vi "Main - Menu Button Ref FGV.vi"(7 "Action":T1=enum."Write", 8 "error In":errorcluster, 11 "Menu Button Ref In":refnum<vi>[](array[refnum])) -> (0 "error out":errorcluster, 3 "Menu Button Ref Out":refnum<vi>[](array[refnum]))   [LabVIEW 2019]
uses:
  Controls/FGV States.ctl
panel:
  # "report\nzero\nhome\nsetting\nmanual\nload\nstop\nstart"
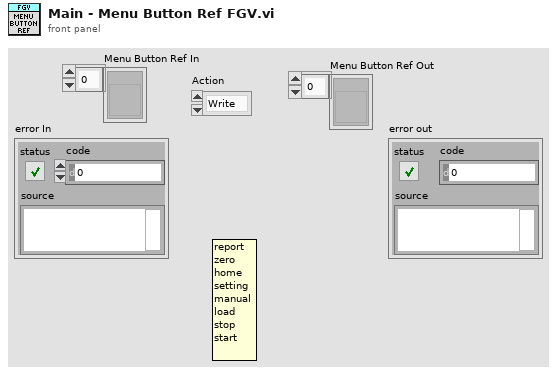
[diagram p1: front panel]
types:
  T1 = typedef "FGV States.ctl" = enum16{"Read", "Write"}
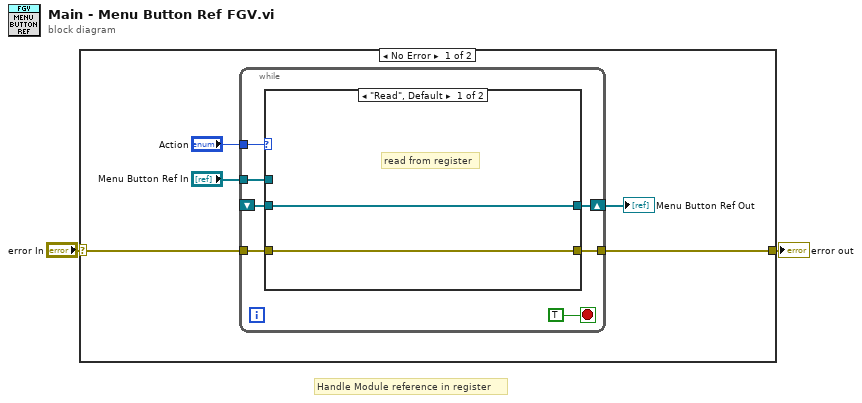
[diagram p0: block diagram]
diagram:
  # "Handle Module reference in register"
  n1 = case shown="No Error" "error In" {
    selector: "error In" -> [w6 w19]
    tunnel: [w5 w19] -> w1
    frame No Error {
      n2 = while {
        tunnel: "Action" -> [w14]
        tunnel: "Menu Button Ref In" -> [w11]
        shift-right: [w12] -> w3
        shift-left: _ -> [w10]
        tunnel: [w9] -> w5
        tunnel: w6 -> [w8]
        stop <- TRUE stop-if-true
        n3 = case shown="\"Read\", Default" w14 {
          tunnel: [w16 w18] -> w12
          tunnel: w11 -> [_ w18]
          tunnel: w10 -> [w16 _]
          tunnel: [w15 w17] -> w9
          tunnel: w8 -> [w15 w17]
          frame "Read", Default {
            # "read from register"
          }
          frame "Write" {
            # "write to register"
          }
        }
      }
      "Menu Button Ref Out" <- w3
    }
    frame Error {
    }
  }
  "error out" <- w1
